vi "Init Device.vi"(8 "error in (no error)":errorcluster, 11 "cetoni in":refnum<class "PHD Ultra.lvclass">) -> (0 "error out":errorcluster, 3 "cetoni out":refnum<class "PHD Ultra.lvclass">)   [LabVIEW 2018, in "PHD Ultra.lvlib" / "PHD Ultra.lvclass"]
uses:
  PHD Ultra.lvclass
  PHD Ultra.lvclass/PHD Ultra.ctl
  Device/Device.lvclass
  <userlib>/QmixLib/QmixLib.lvlib
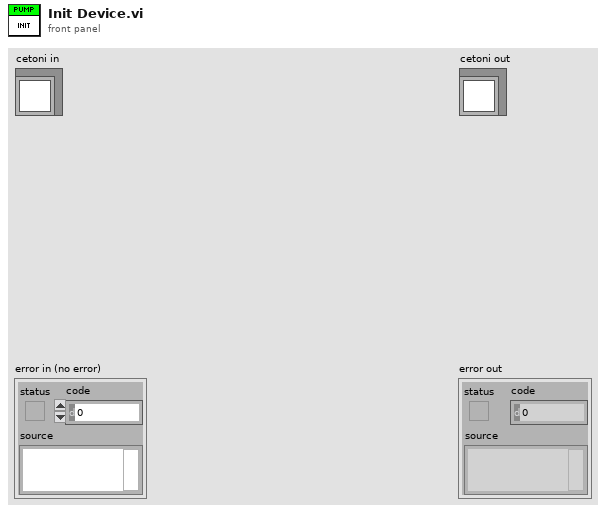
[diagram p1: front panel]
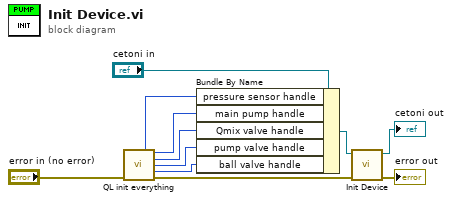
[diagram p0: block diagram]
diagram:
  n1 = call <userlib>:"QL init everything.vi"("error in (no error)"="error in (no error)") -> ("pPressureSensor out"=w7:i64, "pMainPump out"=w4:i64, "pQmixValve out"=w5:i64, "pPumpValve out"=w3:i64, "pBallValve out"=w2:i64, "error out"=w9:errorcluster)  [unwired: 9 in]
  n2 = Bundle By Name(cluster="cetoni in", "pressure sensor handle"=w7, "main pump handle"=w4, "Qmix valve handle"=w5, "pump valve handle"=w3, "ball valve handle"=w2) -> (w6:refnum<class "PHD Ultra.lvclass">)
  n3 = call-parent "Init Device.vi"("error in (no error)"=w9, "Device in"=w6) -> ("error out"=→"error out":errorcluster, "Device out"=→"cetoni out":refnum<class "PHD Ultra.lvclass">)  [unwired: 8 in]
